vi "Actor Core.vi"(8 "error in":errorcluster, 11 "Nested in":refnum<class "demo.lvclass">) -> (0 "error out":errorcluster, 3 "Actor out":refnum<class "Actor.lvclass">)   [LabVIEW 2025, in "demo.lvlib" / "demo.lvclass"]
doc: "(<B>Filename</B>: Actor Framework.lvlib:Actor.lvclass:Actor Core.vi)\n\nReceives messages to the actor, reacts to them, and initiates any error handling that may shut the actor down.\n\nDescendant classes may override this VI to append parallel tasks for the actor to complete while it handles messages. Overrides use the Call Parent Method node."
uses:
  demo.lvclass
  <vilib>/ActorFramework/Actor/Actor.lvclass
  Demo_States/Demo_States/Demo_States.lvclass
  <vilib>/ActorFramework/Actor/Actor.lvclass/Actor.ctl
  <vilib>/ActorFramework/Message Enqueuer/Message Enqueuer.lvclass/Message Enqueuer.ctl
  demo.lvclass/demo.ctl
  <vilib>/ActorFramework/Message Enqueuer/Init from Existing Queue.vi
  <vilib>/ActorFramework/Message Enqueuer/Enqueue.vi
  Demo_States/Demo_States Messages/Go_to_Init Msg/Go_to_Init Msg.lvclass
  Demo_States/Demo_States Messages/Go_to_Login Msg/Go_to_Login Msg.lvclass
  Demo_States/Demo_States Messages/Go_to_State3 Msg/Go_to_State3 Msg.lvclass
  <vilib>/ActorFramework/Stop Msg/Stop Msg.lvclass
  <vilib>/ActorFramework/Message Priority Queue/Priority Enqueue.vi
  <vilib>/ActorFramework/Message Enqueuer/Message Enqueuer.lvclass
panel:
  in  "State3":bool
  in  "Login":bool
  out "State":string
  in  "Init":bool
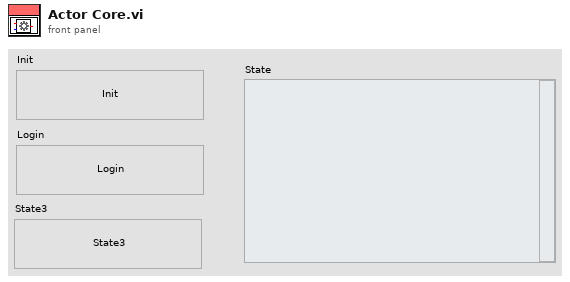
[diagram p1: front panel]
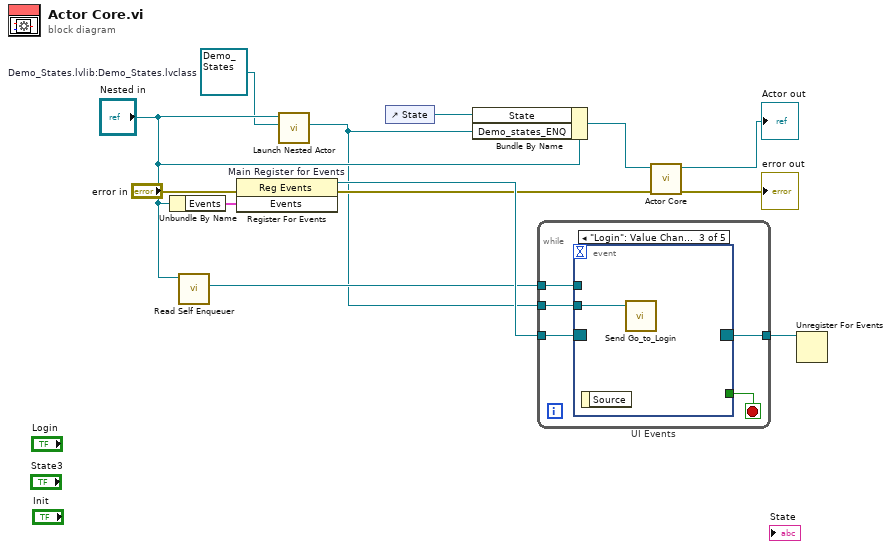
[diagram p0: block diagram]
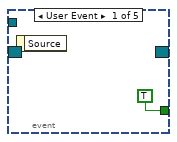
[diagram p2: hidden frame]
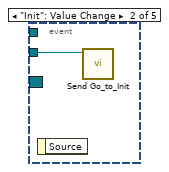
[diagram p3: hidden frame]
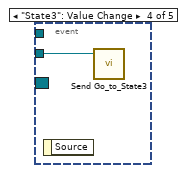
[diagram p4: hidden frame]
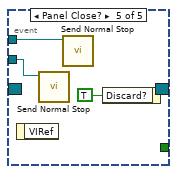
[diagram p5: hidden frame]
diagram:
  w4 = refnum<class "Demo_States.lvclass"> refnum  # Demo_States.lvlib:Demo_States.lvclass
  n1 = Unbundle By Name("Nested in") -> ("Events"=w10:cluster{"Stop":refnum<user-event>})
  n2 = call <vilib>:"Read Self Enqueuer.vi"("Actor"="Nested in") -> ("Self Enqueuer"=w8:refnum<class "Message Enqueuer.lvclass">)  [unwired: 10 in]
  n3 = register-events "Main Register for Events"(error in="error in", w10) -> (reference out=w11:refnum<event-registration>, error out=w6:errorcluster)  [unwired: 1 in]
  n4 = call <vilib>:"Launch Nested Actor.vi"("Nested Actor"=w4, "Caller Actor in"="Nested in") -> ("Nested Actor's Enqueuer"=w1:refnum<class "Message Enqueuer.lvclass">)  [unwired: 7 in, 2 out]
  n5 = control-ref of="State"() -> (w2:refnum<vi>)
  n6 = Bundle By Name(cluster="Nested in", "State"=w2, "Demo_states_ENQ"=w1) -> (w3:refnum<class "demo.lvclass">)
  n7 = while {
    tunnel: w11 -> [w18]
    tunnel: [w16] -> w9
    tunnel: w8 -> [w15]
    tunnel: w1 -> [w14]
    stop <- w17 stop-if-true
    n8 = event "UI Events" shown="[2] \"Login\": Value Change" {
      selector: w18 -> [_ _ _ _ _]
      dyn-events: [_ _ _ _ _] -> w16
      timeout: _ -> [_ _ _ _ _]
      tunnel: [TRUE _ _ _ _] -> w17
      tunnel: w15 -> [_ _ _ _ w24]
      tunnel: w14 -> [_ w20 w21 w22 w23]
      event User Event {
        n9 = event-data() -> ()  [unwired: 1 in, 1 out]
      }
      event "Init": Value Change {
        n10 = event-data() -> ()  [unwired: 1 in, 1 out]
        n11 = call "Send Go_to_Init.vi"("Message Enqueuer"=w20) -> ()  [unwired: 9 in, 2 out]
      }
      event "Login": Value Change {
        n12 = event-data() -> ()  [unwired: 1 in, 1 out]
        n13 = call "Send Go_to_Login.vi"("Message Enqueuer"=w21) -> ()  [unwired: 9 in, 2 out]
      }
      event "State3": Value Change {
        n14 = event-data() -> ()  [unwired: 1 in, 1 out]
        n15 = call "Send Go_to_State3.vi"("Message Enqueuer"=w22) -> ()  [unwired: 9 in, 2 out]
      }
      event Panel Close? {
        n16 = event-data() -> ()  [unwired: 1 in, 1 out]
        n17 = call <vilib>:"Send Normal Stop.vi"("Message Enqueuer"=w23) -> ()  [unwired: 10 in, 1 out]
        n18 = call <vilib>:"Send Normal Stop.vi"("Message Enqueuer"=w24) -> ()  [unwired: 10 in, 1 out]
        n19 = event-data("Discard?"=TRUE) -> ()  [unwired: 1 in, 1 out]
      }
    }
  }
  n20 = call-parent "Actor Core.vi"("error in"=w6, "Actor in"=w3) -> ("error out"=→"error out":errorcluster, "Actor out"=→"Actor out":refnum<class "Actor.lvclass">)  [unwired: 8 in]
  n21 = Unregister For Events(event registration refnum=w9) -> ()  [unwired: 1 in, 1 out]
